vi "Digital Reversed Order.vi"   [LabVIEW 2017, in "NI_AAL_SignalOperation.lvlib"]
doc: "Modifies the input array according to the digital-reversed order of the index."
uses:
  <vilib>/Analysis/NI_AAL_SignalOperation.lvlib
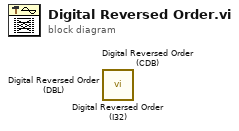
[diagram p0: block diagram]
diagram:
  n1 = call <vilib>:"Digital Reversed Order (I32).vi"() -> ()  [unwired: 9 in, 3 out]
  n2 = call <vilib>:"Digital Reversed Order (CDB).vi"() -> ()  [unwired: 9 in, 3 out]
  n3 = call <vilib>:"Digital Reversed Order (DBL).vi"() -> ()  [unwired: 9 in, 3 out]
